vi "writetable.vi"(7 "std sample":T1(array[cluster]), 8 "col":i32, 9 "Array in":dbl[](array[numeric]), 10 "type":i32, 11 "reference":refnum<vi>) -> ()   [LabVIEW 2013]
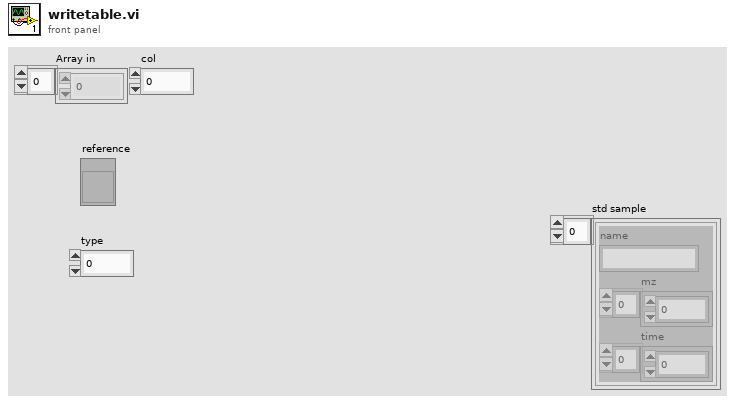
[diagram p1: front panel]
types:
  T1 = cluster{"name":string, "mz":dbl[], "time":dbl[]}[]
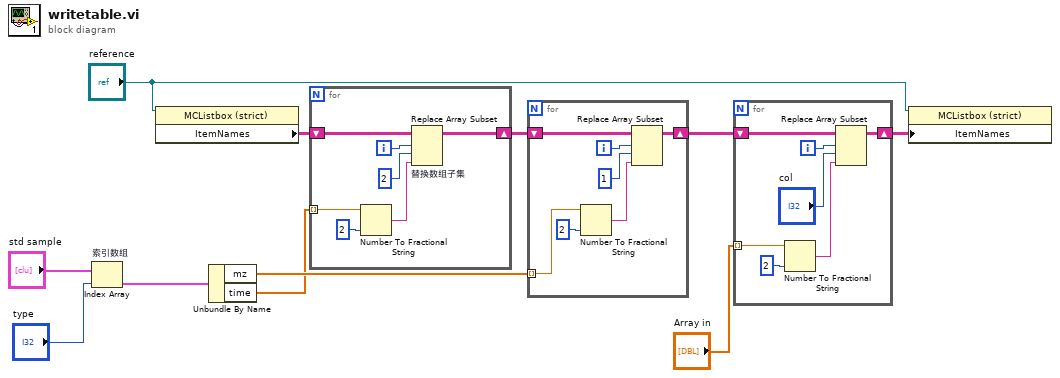
[diagram p0: block diagram]
diagram:
  n1 = Index Array "索引数组"(array="std sample", index="type") -> (element=w9:cluster{"name":string, "mz":dbl[], "time":dbl[]})
  n2 = property on="Property Node" class="MCListbox (strict)"(reference="reference") -> ("ItemNames"=w2:string[][])  [unwired: 1 in, 2 out]
  n3 = Unbundle By Name(w9) -> ("mz"=w8:dbl[], "time"=w3:dbl[])
  n4 = for {
    tunnel: w3 -> [w16] mode=indexing
    shift-right: [w15] -> w1
    shift-left: w2 -> [w18]
    i -> [w17]
    n5 = Number To Fractional String(number=w16, precision (6)=i16 2) -> (F-format string=w14:string)  [unwired: 2 in]
    n6 = Replace Array Subset "替换数组子集"(array=w18, new element=w14, index (row)=w17, index (col)=2 ("disabled index (col)")) -> (w15:string[][])
  }
  n7 = for {
    tunnel: w8 -> [w23] mode=indexing
    shift-right: [w22] -> w7
    shift-left: w1 -> [w25]
    i -> [w24]
    n8 = Number To Fractional String(number=w23, precision (6)=i16 2) -> (F-format string=w21:string)  [unwired: 2 in]
    n9 = Replace Array Subset(array=w25, new element=w21, index (row)=w24, index (col)=1 ("disabled index (col)")) -> (w22:string[][])
  }
  n10 = for {
    shift-right: [w27] -> w5
    shift-left: w7 -> [w32]
    tunnel: "Array in" -> [w29] mode=indexing
    i -> [w31]
    n11 = Number To Fractional String(number=w29, precision (6)=i16 2) -> (F-format string=w28:string)  [unwired: 2 in]
    n12 = Replace Array Subset(array=w32, new element=w28, index (row)=w31, index (col)="col") -> (w27:string[][])
  }
  n13 = property on="Property Node" class="MCListbox (strict)"(reference="reference", "ItemNames"=w5) -> ()  [unwired: 1 in, 2 out]
